vi "Teleop.vi"(10 "Match Info":T1={"Autonomous Elapsed Seconds"=0.0, "TeleOp Elapsed Seconds"=0.0, "Disabled Elapsed Seconds"=0.0, "Visited Autonomous"=FALSE, "Visited TeleOp"=FALSE, "Visited Disabled"=FALSE, "Autonomous Settings"={"Autonomous Style"=enum."Independent", "VI Refnum"=refnum}}, 11 "Call Context":T2) -> ()   [LabVIEW 2017]
doc: "This VI is called for each TeleOp packet received from the DS where the robot is not disabled. It is often used to read from the joysticks and update I/O or to update setpoints for timed control loops. It should complete and return within 20 milliseconds or it may miss DS packets."
uses:
  <vilib>/Rock Robotics/WPI/DriverStation/WPI_DriverStationDerivedRobotMode.ctl
  <vilib>/Rock Robotics/WPI/DriverStation/WPI_DriverStationMatch Info.ctl
  <vilib>/Rock Robotics/Network Tables/NT Read Boolean.vi
  <vilib>/Rock Robotics/Network Tables/NT Read Number.vi
  <vilib>/Rock Robotics/WPI/Utilities/WPI_GetSetVariantRefNum.vi
  <vilib>/Rock Robotics/Network Tables/NT Write Boolean Array.vi
  <vilib>/Rock Robotics/Network Tables/NT Write Numeric Array.vi
  Robot Global Data.vi
panel:
  out "Sample Slider 0":dbl(slide) scale=0.0..5.0
  out "Sample Boolean 1":bool
  out "Sample Boolean 0":bool
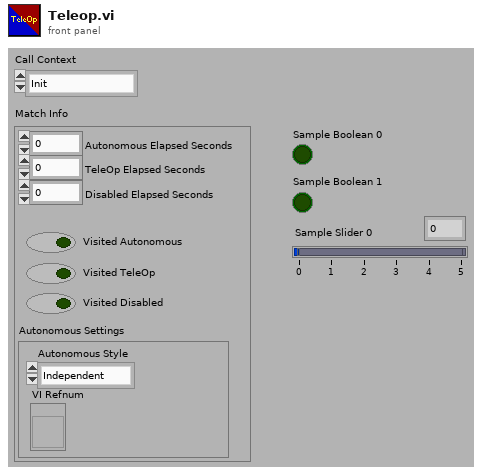
[diagram p1: front panel]
types:
  T1 = typedef "WPI_DriverStationMatch Info.ctl" = cluster{"Autonomous Elapsed Seconds":dbl, "TeleOp Elapsed Seconds":dbl, "Disabled Elapsed Seconds":dbl, "Visited Autonomous":bool, "Visited TeleOp":bool, "Visited Disabled":bool, "Autonomous Settings":cluster{"Autonomous Style":enum16{"Iterative", "Independent"}, "VI Refnum":refnum<vi>}}
  T2 = typedef "WPI_DriverStationDerivedRobotMode.ctl" = enum16{"Init", "Execute", "Stop"}
  T3 = typedef "WPI_JoystickDevRef.ctl" = cluster{"Device":T4}
  T4 = typedef "WPI_JoystickDeviceEnum.ctl" = enum16{"USB 0", "USB 1", "USB 2", "USB 3", "USB 4", "USB 5"}
  T5 = cluster{"Axes[0]":dbl, "Axes[1]":dbl, "Axes[2]":dbl, "Axes[3]":dbl, "Axes[4]":dbl, "Axes[5]":dbl, "Axes[6]":dbl, "Axes[7]":dbl, "Axes[8]":dbl}
  T6 = cluster{"Buttons[0]":bool, "Buttons[1]":bool, "Buttons[2]":bool, "Buttons[3]":bool, "Buttons[4]":bool, "Buttons[5]":bool, "Buttons[6]":bool, "Buttons[7]":bool, "Buttons[8]":bool}
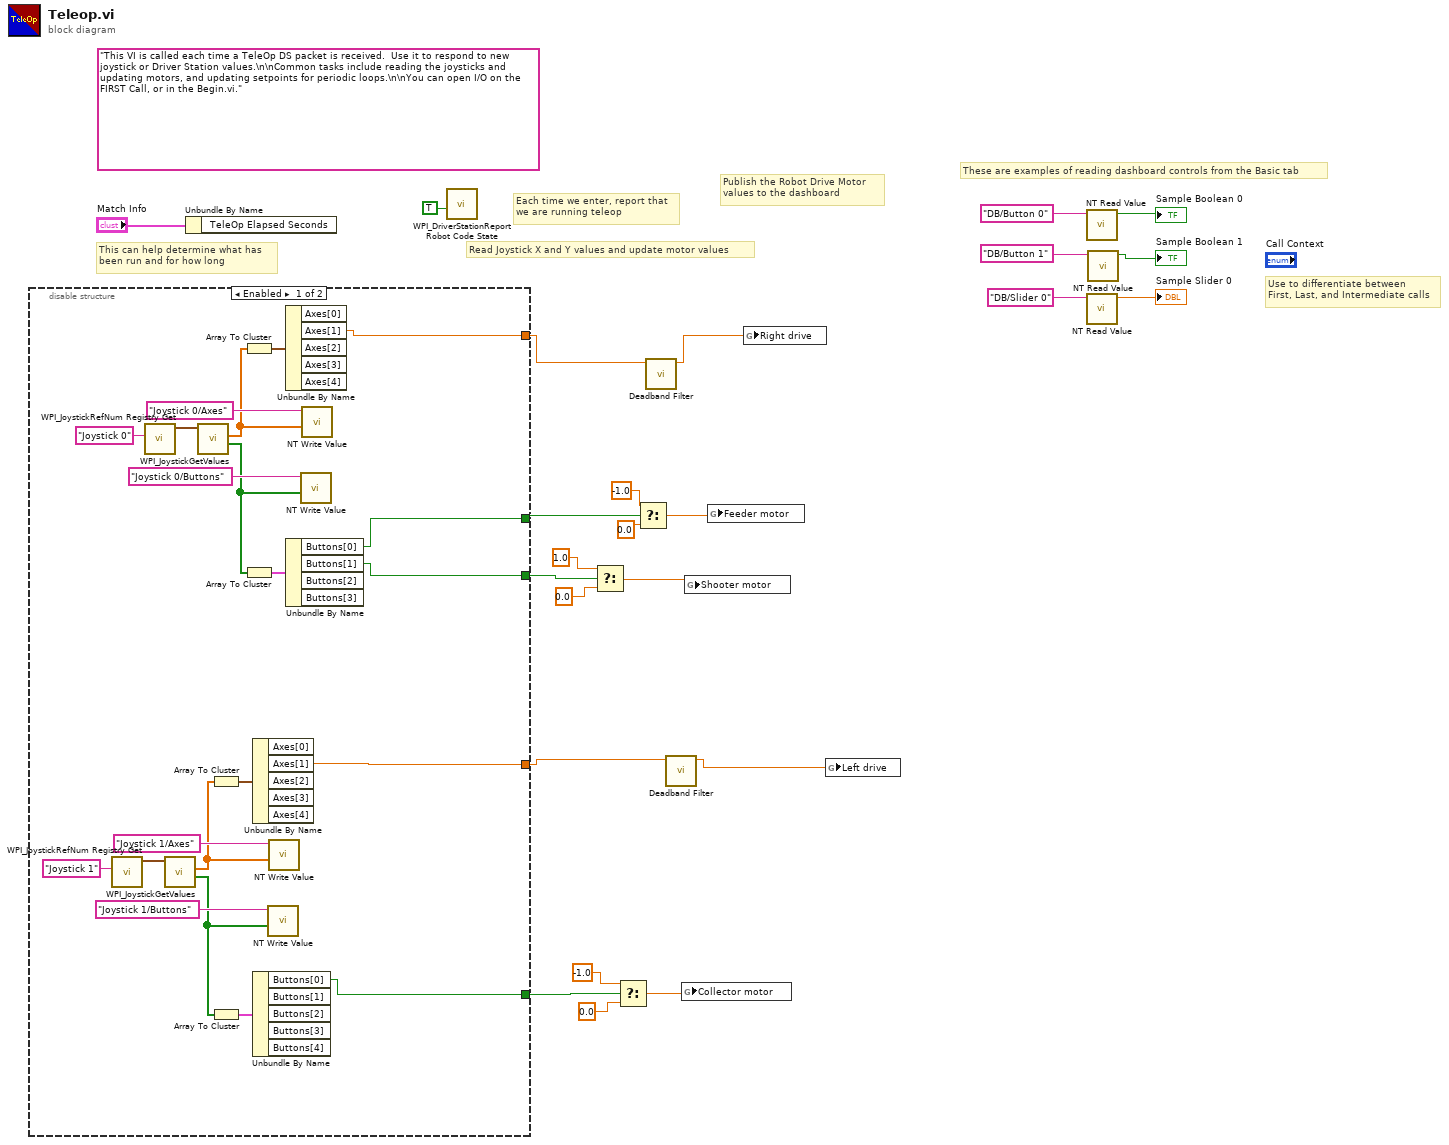
[diagram p0: block diagram]
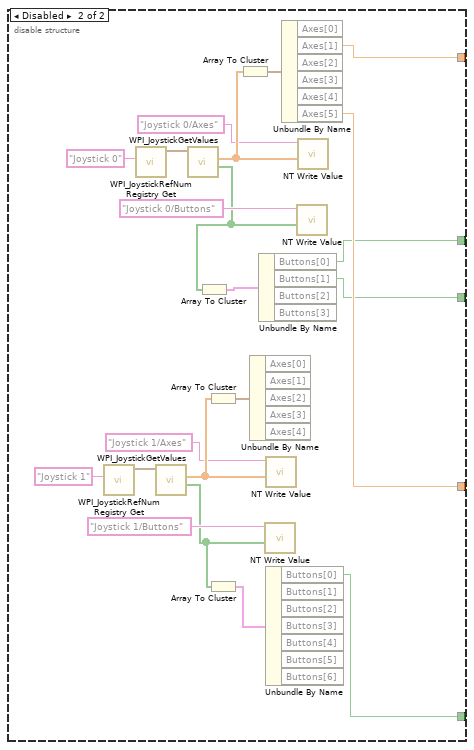
[diagram p2: hidden frame]
diagram:
  (unwired) "This VI is called each time a TeleOp DS packet is received.  Use it to respond to new joystick or Driver Station values.\n\nCommon tasks include reading the joysticks and updating motors, and updating setpoints for periodic loops.\n\nYou can open I/O on the FIRST Call, or in the Begin.vi."
  # "These are examples of reading dashboard controls from the Basic tab"
  # "Publish the Robot Drive Motor\nvalues to the dashboard"
  # "Each time we enter, report that\nwe are running teleop"
  # "Use to differentiate between\nFirst, Last, and Intermediate calls"
  # "This can help determine what has\nbeen run and for how long"
  # "Read Joystick X and Y values and update motor values"
  n1 = disable-structure shown="Enabled" {
    disable-tunnel: [w25 w54] -> w4
    disable-tunnel: [w33 w53] -> w2
    disable-tunnel: [w28 w48] -> w16
    disable-tunnel: [w27 w47] -> w5
    disable-tunnel: [w26 w46] -> w6
    frame Enabled {
      n2 = call <vilib>:"WPI_JoystickRefNum Registry Get.vi"("refnum name"="Joystick 1") -> ("JoystickDevRef"=w38:T3)  [unwired: 1 in, 9 out]
      n3 = call <vilib>:"WPI_JoystickRefNum Registry Get.vi"("refnum name"="Joystick 0") -> ("JoystickDevRef"=w44:T3)  [unwired: 1 in, 9 out]
      n4 = call <vilib>:"WPI_JoystickGetValues.vi"("JoystickDevRef"=w38) -> ("Buttons"=w30:bool[], "Axes"=w35:dbl[])  [unwired: 6 in, 3 out]
      n5 = call <vilib>:"WPI_JoystickGetValues.vi"("JoystickDevRef"=w44) -> ("Buttons"=w32:bool[], "Axes"=w41:dbl[])  [unwired: 6 in, 3 out]
      n6 = Array To Cluster(array=w35) -> (cluster=w34:T5)
      n7 = Array To Cluster(array=w30) -> (cluster=w29:T6)
      n8 = Array To Cluster(array=w41) -> (cluster=w40:T5)
      n9 = Array To Cluster(array=w32) -> (cluster=w31:T6)
      n10 = Unbundle By Name(w34) -> ("Axes[1]"=w33:dbl)  [unwired: 4 out]
      n11 = Unbundle By Name(w29) -> ("Buttons[0]"=w28:bool)  [unwired: 4 out]
      n12 = call-poly <vilib>:"NT Write Value.vi"("Boolean Array"=w30, "Name"="Joystick 1/Buttons") -> ()  [unwired: 9 in, 1 out]
      n13 = call-poly <vilib>:"NT Write Value.vi"("Numeric Array"=w35, "Name"="Joystick 1/Axes") -> ()  [unwired: 9 in, 1 out]
      n14 = Unbundle By Name(w40) -> ("Axes[1]"=w25:dbl)  [unwired: 4 out]
      n15 = Unbundle By Name(w31) -> ("Buttons[0]"=w26:bool, "Buttons[1]"=w27:bool)  [unwired: 2 out]
      n16 = call-poly <vilib>:"NT Write Value.vi"("Boolean Array"=w32, "Name"="Joystick 0/Buttons") -> ()  [unwired: 9 in, 1 out]
      n17 = call-poly <vilib>:"NT Write Value.vi"("Numeric Array"=w41, "Name"="Joystick 0/Axes") -> ()  [unwired: 9 in, 1 out]
    }
    frame Disabled {
      n18 = call <vilib>:"WPI_JoystickRefNum Registry Get.vi"("refnum name"="Joystick 1") -> ("JoystickDevRef"=w64:T3)  [unwired: 1 in, 9 out]
      n19 = call <vilib>:"WPI_JoystickRefNum Registry Get.vi"("refnum name"="Joystick 0") -> ("JoystickDevRef"=w61:T3)  [unwired: 1 in, 9 out]
      n20 = call <vilib>:"WPI_JoystickGetValues.vi"("JoystickDevRef"=w64) -> ("Buttons"=w50:bool[], "Axes"=w65:dbl[])  [unwired: 6 in, 3 out]
      n21 = call <vilib>:"WPI_JoystickGetValues.vi"("JoystickDevRef"=w61) -> ("Buttons"=w52:bool[], "Axes"=w62:dbl[])  [unwired: 6 in, 3 out]
      n22 = Array To Cluster(array=w52) -> (cluster=w51:T6)
      n23 = Array To Cluster(array=w65) -> (cluster=w66:T5)
      n24 = Array To Cluster(array=w50) -> (cluster=w49:T6)
      n25 = Array To Cluster(array=w62) -> (cluster=w63:T5)
      n26 = Unbundle By Name(w66) -> ()  [unwired: 5 out]
      n27 = Unbundle By Name(w51) -> ("Buttons[0]"=w46:bool, "Buttons[1]"=w47:bool)  [unwired: 2 out]
      n28 = call-poly <vilib>:"NT Write Value.vi"("Boolean Array"=w50, "Name"="Joystick 1/Buttons") -> ()  [unwired: 9 in, 1 out]
      n29 = call-poly <vilib>:"NT Write Value.vi"("Numeric Array"=w65, "Name"="Joystick 1/Axes") -> ()  [unwired: 9 in, 1 out]
      n30 = Unbundle By Name(w49) -> ("Buttons[0]"=w48:bool)  [unwired: 6 out]
      n31 = Unbundle By Name(w63) -> ("Axes[1]"=w54:dbl, "Axes[5]"=w53:dbl)  [unwired: 4 out]
      n32 = call-poly <vilib>:"NT Write Value.vi"("Boolean Array"=w52, "Name"="Joystick 0/Buttons") -> ()  [unwired: 9 in, 1 out]
      n33 = call-poly <vilib>:"NT Write Value.vi"("Numeric Array"=w62, "Name"="Joystick 0/Axes") -> ()  [unwired: 9 in, 1 out]
    }
  }
  n34 = Unbundle By Name("Match Info") -> ()  [unwired: 1 out]
  n35 = call <vilib>:"WPI_DriverStationReport Robot Code State.vi"("TeleOp"=TRUE ("Autonomous")) -> ()  [unwired: 10 in, 1 out]
  n36 = Select(t=1.0, s=w5, f=0.0) -> (s? t:f=w10:dbl)
  n37 = Select(t=-1.0, s=w16, f=0.0) -> (s? t:f=w13:dbl)
  n38 = Select(t=-1.0, s=w6, f=0.0) -> (s? t:f=w7:dbl)
  n39 = call "Deadband Filter.vi"("Joystick axis"=w4) -> ("Filtered axis"=w3:dbl)  [unwired: 10 in]
  n40 = call "Deadband Filter.vi"("Joystick axis"=w2) -> ("Filtered axis"=w1:dbl)  [unwired: 10 in]
  n41 = global write "Robot Global Data.vi" "Collector motor"(w13) -> ()
  n42 = global write "Robot Global Data.vi" "Shooter motor"(w10) -> ()
  n43 = global write "Robot Global Data.vi" "Feeder motor"(w7) -> ()
  n44 = global write "Robot Global Data.vi" "Right drive"(w3) -> ()
  n45 = global write "Robot Global Data.vi" "Left drive"(w1) -> ()
  n46 = call-poly <vilib>:"NT Read Value.vi"("Name"="DB/Button 0" ("refnum name")) -> ("Boolean"=→"Sample Boolean 0":bool)  [unwired: 9 in, 1 out]
  n47 = call-poly <vilib>:"NT Read Value.vi"("Name"="DB/Slider 0" ("refnum name")) -> ("Numeric"=→"Sample Slider 0":dbl)  [unwired: 9 in, 1 out]
  n48 = call-poly <vilib>:"NT Read Value.vi"("Name"="DB/Button 1" ("refnum name")) -> ("Boolean"=→"Sample Boolean 1":bool)  [unwired: 9 in, 1 out]
